vi "Slave3.vi"() -> ()   [LabVIEW 2012]
uses:
  MyGlobals.vi
panel:
  out "Slave3Text":string
  in  "Slave3 Original":string="Is"
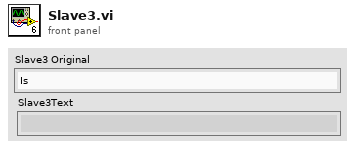
[diagram p1: front panel]
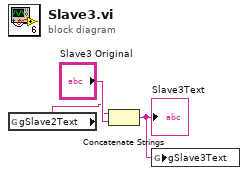
[diagram p0: block diagram]
diagram:
  n1 = global read "MyGlobals.vi" "gSlave2Text"() -> (w1:string)
  n2 = Concatenate Strings(w1, "Slave3 Original") -> (w3:string)
  "Slave3Text" <- w3
  n3 = global write "MyGlobals.vi" "gSlave3Text"(w3) -> ()
